vi "Trigger Selection Display.vi"(8 "error in (no error)":errorcluster, 11 "reference":refnum<vi>) -> (0 "error out":errorcluster)   [LabVIEW 2020, in "Settings Editor.lvlib"]
uses:
  Settings Editor.lvlib
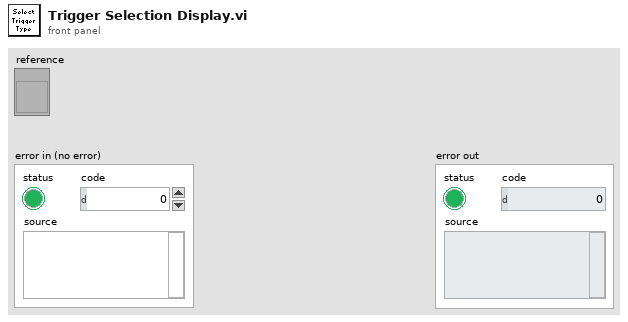
[diagram p1: front panel]
types:
  T1 = typedef "Settings Editor.lvlib/DAQmx Trigger Settings--cluster.ctl" = cluster{"Trigger Type":enum32{"No Trigger", "Digital Start", "Digital Pause", "Digital Reference", "Analog Start", "Analog Pause", "Analog Reference", "Time Start"}, "Digital Start":cluster{"Source":tag, "Digital Start Trigger Edge":i32}, "Digital Pause":cluster{"Source":tag, "Digital Pause Trigger Pause When":i32}, "Digital Reference":cluster{"DAQmx Terminal":tag, "Digital Start Trigger Edge":i32, "Digital Reference Pretrigger Samples":u32}, "Analog Start":cluster{"Source":string, "Digital Start Trigger Edge":i32, "Analog Start Trigger Hysteresis":dbl, "Analog Start Trigger Level":dbl}, "Analog Pause":cluster{"Source":string, "Analog Start Trigger Level":dbl, "Analog Pause Trigger Pause When":i32}, "Analog Reference":cluster{"Source":string, "Digital Start Trigger Edge":i32, "Analog Start Trigger Hysteresis":u32, "Analog Start Trigger Level":dbl}, "Time Start":cluster{"Select Time\nManually":bool, "When":timestamp}}
  T2 = enum32{"No Trigger", "Digital Start", "Digital Pause", "Digital Reference", "Analog Start", "Analog Pause", "Analog Reference", "Time Start"}
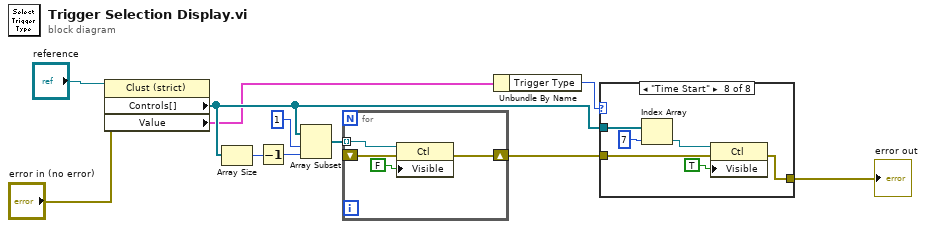
[diagram p0: block diagram]
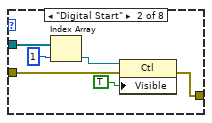
[diagram p3: hidden frame]
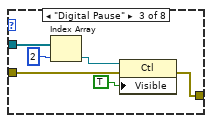
[diagram p4: hidden frame]
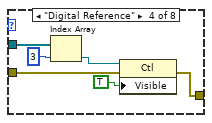
[diagram p5: hidden frame]
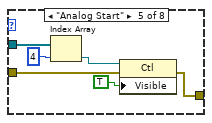
[diagram p6: hidden frame]
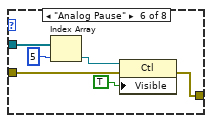
[diagram p7: hidden frame]
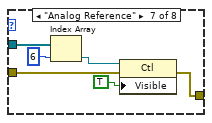
[diagram p8: hidden frame]
diagram:
  n1 = property class="Clust (strict)"(reference="reference", error in="error in (no error)") -> ("Controls[]"=w7:refnum<vi>[], "Value"=w2:T1)  [unwired: 2 out]
  n2 = Array Size(array=w7) -> (size(s)=w6:i32)
  n3 = Decrement(x=w6) -> (x-1=w5:i32)
  n4 = Array Subset(array=w7, index=1, length=w5) -> (w9:refnum<vi>[])
  n5 = for {
    tunnel: w9 -> [w14] mode=indexing
    shift-right: [w12] -> w10
    shift-left: _ -> [w15]
    n6 = property class="Ctl"(reference=w14, error in=w15, "Visible"=FALSE) -> (error out=w12:errorcluster)  [unwired: 1 out]
  }
  n7 = Unbundle By Name(w2) -> ("Trigger Type"=w11:T2)
  n8 = case shown="\"Time Start\"" w11 {
    tunnel: w7 -> [_ w18 w25 w31 w37 w43 w49 w55]
    tunnel: w10 -> [w16 w19 w24 w30 w36 w42 w48 w54]
    tunnel: [w16 w17 w23 w29 w35 w41 w47 w53] -> w3
    frame "No Trigger", Default {
    }
    frame "Digital Start" {
      n9 = Index Array(array=w18, index=1) -> (element=w22:refnum<vi>)
      n10 = property class="Ctl"(reference=w22, error in=w19, "Visible"=TRUE) -> (error out=w17:errorcluster)  [unwired: 1 out]
    }
    frame "Digital Pause" {
      n11 = Index Array(array=w25, index=2) -> (element=w28:refnum<vi>)
      n12 = property class="Ctl"(reference=w28, error in=w24, "Visible"=TRUE) -> (error out=w23:errorcluster)  [unwired: 1 out]
    }
    frame "Digital Reference" {
      n13 = Index Array(array=w31, index=3) -> (element=w34:refnum<vi>)
      n14 = property class="Ctl"(reference=w34, error in=w30, "Visible"=TRUE) -> (error out=w29:errorcluster)  [unwired: 1 out]
    }
    frame "Analog Start" {
      n15 = Index Array(array=w37, index=4) -> (element=w40:refnum<vi>)
      n16 = property class="Ctl"(reference=w40, error in=w36, "Visible"=TRUE) -> (error out=w35:errorcluster)  [unwired: 1 out]
    }
    frame "Analog Pause" {
      n17 = Index Array(array=w43, index=5) -> (element=w46:refnum<vi>)
      n18 = property class="Ctl"(reference=w46, error in=w42, "Visible"=TRUE) -> (error out=w41:errorcluster)  [unwired: 1 out]
    }
    frame "Analog Reference" {
      n19 = Index Array(array=w49, index=6) -> (element=w52:refnum<vi>)
      n20 = property class="Ctl"(reference=w52, error in=w48, "Visible"=TRUE) -> (error out=w47:errorcluster)  [unwired: 1 out]
    }
    frame "Time Start" {
      n21 = Index Array(array=w55, index=7) -> (element=w58:refnum<vi>)
      n22 = property class="Ctl"(reference=w58, error in=w54, "Visible"=TRUE) -> (error out=w53:errorcluster)  [unwired: 1 out]
    }
  }
  "error out" <- w3
